vi "NonCoherencyWindowing.vi"() -> ()   [LabVIEW 2009]
uses:
  <vilib>/imath/engines/lvmath2/RunTimeEngine/ErrorHandling/NIMS_Finalize Error.vi
  <vilib>/imath/engines/lvmath2/RunTimeEngine/Parser/MC_Version.vi
  <vilib>/imath/engines/lvmath2/RunTimeEngine/Managers/WorkSpace/UID Generator.vi
  <vilib>/imath/engines/lvmath2/RunTimeEngine/NodeEndStatement/NIMS_NodeEndStatement_Output.vi
  <instcachedir>/0/NIMS_NodeEndStatement_Output_53EC0D466D134D7ABD903AC30B43404B.lvgen/NIMS_NodeEndStatement_Output_53EC0D466D134D7ABD903AC30B43404B_001.vi
  <vilib>/imath/engines/lvmath2/RunTimeEngine/NodeEndStatement/MC_NodeEndStatement_Dispose.vi
  <vilib>/imath/engines/lvmath/Functions/Error Handling/MergeErrorsWrapper.vi
  <vilib>/imathl/engines/lvmath/Functions/Error Handling/Create Error.vi
  <vilib>/imath/engines/lvmath2/RunTimeEngine/RunTimeType/NIMS_RunTimeType_Get Case Value.vi
  <vilib>/imath/engines/lvmath2/RunTimeEngine/Managers/SymbolTable/Read Variable.vi
  <vilib>/imath/engines/lvmath2/RunTimeEngine/CommandStatement/NIMS_CommandStatement_MaskErr.vi
  <vilib>/imath/engines/lvmath2/RunTimeEngine/Managers/SymbolTable/Write Variable.vi
  <vilib>/imath/engines/lvmath2/RunTimeEngine/RunTimeSymbolToken/NIMS_RunTimeSymbolToken_ResolveUDForVariable.vi
  <vilib>/imath/engines/lvmath2/RunTimeEngine/RangeToken/NIMS_NS_Range - 2 inputs.vi
  <vilib>/imath/engines/lvmath2/RunTimeEngine/ArithmeticOperatorToken/NIMS_NS_ArithmeticOperator_rightdivmx.vi
  <vilib>/imath/engines/lvmath2/RunTimeEngine/RunTimeSymbolToken/NIMS_RunTimeSymbolToken_ReadVariable.vi
  <vilib>/imath/engines/lvmath2/RunTimeEngine/ArithmeticOperatorToken/NIMS_NS_ArithmeticOperator_multmx.vi
  <vilib>/imath/engines/lvmath2/RunTimeEngine/RunTimeSymbolToken/NIMS_RunTimeSymbolToken_ResolveSymbol.vi
  <instcachedir>/0/NIMS_RunTimeSymbolToken_ResolveSymbol_94D143D0F28444E2BA7BB87D83E1A664.lvgen/NIMS_RunTimeSymbolToken_ResolveSymbol_94D143D0F28444E2BA7BB87D83E1A664_000.vi
  <vilib>/imath/engines/lvmath2/RunTimeEngine/ArithmeticOperatorToken/NIMS_NS_ArithmeticOperator_plus.vi
  <vilib>/imath/engines/lvmath2/RunTimeEngine/ArithmeticOperatorToken/NIMS_NS_ArithmeticOperator_minus.vi
  <instcachedir>/0/NIMS_RunTimeSymbolToken_ResolveSymbol_94D143D0F28444E2BA7BB87D83E1A664.lvgen/NIMS_RunTimeSymbolToken_ResolveSymbol_94D143D0F28444E2BA7BB87D83E1A664_001.vi
  <vilib>/imath/engines/lvmath2/RunTimeEngine/RunTimeType/NIMS_RunTimeType_From StrictType (excl LVString).vi
  <vilib>/imath/engines/lvmath2/RunTimeEngine/NonStaticBuiltInFunctions/Manual/NIMS_NS_global.vi
  <vilib>/imath/engines/lvmath2/RunTimeEngine/NonStaticBuiltInFunctions/NIMS_NS_cos.vi
  <vilib>/imath/engines/lvmath2/RunTimeEngine/NonStaticBuiltInFunctions/NIMS_NS_fft.vi
  <vilib>/imath/engines/lvmath2/RunTimeEngine/NonStaticBuiltInFunctions/NIMS_NS_abs.vi
  <vilib>/imath/engines/lvmath2/RunTimeEngine/NonStaticBuiltInFunctions/NIMS_NS_log10.vi
  <vilib>/imath/engines/lvmath2/RunTimeEngine/NodeEndStatement/NIMS_NodeEndStatement_Get Vector.vi
  <instcachedir>/0/NIMS_NodeEndStatement_Get Vector_708AE642CFEE4B9892E482CBBBA3A4D6.lvgen/NIMS_NodeEndStatement_Get Vector_708AE642CFEE4B9892E482CBBBA3A4D6_001.vi
  <vilib>/imath/engines/lvmath2/RunTimeEngine/RunTimeType/NIMS_RunTimeType_To Numeric.vi
  <instcachedir>/0/NIMS_RunTimeType_To Numeric_461D4BB0B5AC4C7A80E516929E1870C9.lvgen/NIMS_RunTimeType_To Numeric_461D4BB0B5AC4C7A80E516929E1870C9_000.vi
  <vilib>/imath/engines/lvmath/Plug In/_Char/NIMS_CH_Character 1D to U8 1D.vi
  <instcachedir>/0/NIMS_NodeEndStatement_Get Vector_708AE642CFEE4B9892E482CBBBA3A4D6.lvgen/NIMS_NodeEndStatement_Get Vector_708AE642CFEE4B9892E482CBBBA3A4D6_002.vi
  <vilib>/imath/engines/lvmath/Plug In/_Char/RunTimeType/NIMS_CH_RunTimeType_To Character 2D.vi
  <vilib>/imath/engines/lvmath/Functions/Error Handling/error.ctl
  <vilib>/imath/engines/lvmath2/RunTimeEngine/ArithmeticOperatorToken/NIMS_NS_ArithmeticOperator_times.vi
  <vilib>/imath/engines/lvmath2/RunTimeEngine/ArithmeticOperatorToken/NIMS_NS_ArithmeticOperator_cctranspose.vi
  <vilib>/imath/engines/lvmath2/RunTimeEngine/NonStaticBuiltInFunctions/NIMS_NS_win_hann2.vi
  <vilib>/imath/engines/lvmath2/RunTimeEngine/NonStaticBuiltInFunctions/NIMS_NS_freqzd.vi
  <vilib>/imath/engines/lvmath2/RunTimeEngine/NonStaticBuiltInFunctions/NIMS_NS_win_hamming.vi
  <vilib>/imath/engines/lvmath2/RunTimeEngine/NonStaticBuiltInFunctions/NIMS_NS_win_rect.vi
  <vilib>/imath/engines/lvmath2/RunTimeEngine/Managers/SymbolTable/NIMS_WorkSpace.lvlib
panel:
  in  "Tab Control":enum32{"Input Signals", "Windowing Response"}(tab)
  out "Time":dbl[](graph)=[1.0519999999999998, 0.892635758350692, 0.48671366566360336, -0.014213960529799927, -0.48286399816495823, -0.8332750693454192, -0.9844439089484842, -0.8790173197927672, -0.5425141352910673, -0.07907293537832781, 0.39766710213006506, 0.7950512926839483, 1.0127676392121494, 0.9537752599165119, 0.6072435956998912, 0.0922920759743344, -0.41561505518673614, -0.7885340013883491, -0.9648884833134171, -0.911548116681293, -0.6264833485669233, -0.17599282135085542, 0.31594201614569883, 0.7279199339174797, 0.9717386381220531, 0.9789366799794423, 0.7140755998833661, 0.22979152936681138, -0.32102600764294553, -0.76153026470899, -0.979672712648837, -0.9457238312903217, -0.6821570337182414, -0.25169868445329474, 0.2399555283178424, 0.6689028600572418, 0.9344300816682857, 0.9747853105549835, 0.7654072870023012, 0.3376131259459527, -0.19825451970370167, -0.6793358027763582, -0.9634650376378693, -0.9837135532483375, -0.7508142403449144, -0.33382717711029797, 0.1566403020999526, 0.5966924386654645, 0.8876652145787984, 0.9715292169265111, 0.8206100103361844, 0.44487353719016887, -0.07499320335923955, -0.5870694406395051, -0.9326941295433538, -1.019040372240394, -0.8358834391160587, -0.43566821485006507, 0.07592488783600401, 0.5544251498665185, 0.8704100296507408, 0.964260301096264, 0.8383083974973854, 0.5137376584936127, 0.03499999999999957, -0.48585261295939564, -0.8818652804506516, -1.0229561184206226, -0.8845509930676749, -0.5247145097090272, -0.03421866135883577, 0.46859297497064295, 0.840786779414677, 0.9751969639176659, 0.8614359855640242, 0.5601553978306019, 0.1333879750007619, -0.356995848551684, -0.7952068779929633, -1.0252578021844054, -0.9547362823906638, -0.620110912675251, -0.137507594251358, 0.372068182475295, 0.791142680899002, 0.9993468717462828, 0.9279628829910677, 0.6173563155048777, 0.1802855497563253, -0.28407697645575897, -0.702914526162896, -0.9776488534124683, -0.9933831759695436, -0.7139122080215445, -0.23334898138495994, 0.28978814517635426, 0.7221570337182422, 0.9703821129164357, 0.9663755650482756, 0.7004567661150796, 0.2581711069013682, -0.2223730173404324, -0.6324440323293156, -0.9073207446267804, -0.9820539394221334, -0.7966372182568109, -0.36908259607946664, 0.1722255147849101, 0.6557003844606163, 0.9527237315353941, 0.9994814002292728, 0.78509143650267, 0.36268612299860076, -0.14503930774567764, -0.594528329039942, -0.8856811014773216, -0.9710022598166805, -0.8268249390909151, -0.45949731137287486, 0.05406040835925627, 0.5658950662399057, 0.920493181781949, 1.0203444418805658, 0.8458311373029045, 0.4491073291399612, -0.05639584288440221, -0.528310205810283, -0.8499316903093769]
  out "Frequency Domain":dbl[](graph)=[-36.063010068605344, -35.48013279039274, -34.00368270005921, -32.08344281023172, -29.968400742690303, -27.713180557630817, -25.259324216625465, -22.455608089448322, -18.990832409863973, -14.07794602915972, -4.114913838712823, -3.7403821330415536, -12.946788106870805, -17.080106791999548, -19.72637758714805, -21.54183948254877, -23.16627515506536, -24.401566317457796, -25.443897985258722, -26.343781674957675, -24.226903730320053, -27.839889690043492, -28.476824068317693, -29.059155277051325, -29.599056422316544, -30.110000536672633, -30.614092450790913, -31.1765534431675, -32.358923373450644, -30.386487172294476, -29.468348510203928, -31.912759453430546, -32.26618517164874, -32.57308011024947, -32.85063385246029, -33.10613681596499, -33.343474150812, -33.565060432808615, -33.77256514899041, -33.96723171385923, -34.15003564865244, -34.32177087608298, -34.48310064590985, -34.634589628770996, -34.776725291880645, -34.909932813665826, -35.03458590340212, -35.15101490873227, -35.259513056057415, -35.36034136097869, -35.45373256257553, -35.53989432202372, -35.61901185371619, -35.69125010943872, -35.75675560394464, -35.81565794790601, -35.868071138314555, -35.91409464485639, -35.95381432218219, -35.98730317150038, -36.01462196987916, -36.03581978166229, -36.0509343632001, -36.05999246943212]
  out "Window (time domain)":dbl[][](graph)=[[1.0, 1.0, 1.0, 1.0, 1.0, 1.0, 1.0, 1.0, 1.0, 1.0, 1.0, 1.0, 1.0, 1.0, 1.0, 1.0, 1.0, 1.0, 1.0, 1.0, 1.0, 1.0, 1.0, 1.0, 1.0, 1.0, 1.0, 1.0, 1.0, 1.0, 1.0, 1.0, 1.0, 1.0, 1.0, 1.0, 1.0, 1.0, 1.0, 1.0, 1.0, 1.0, 1.0, 1.0, 1.0, 1.0, 1.0, 1.0, 1.0, 1.0, 1.0, 1.0, 1.0, 1.0, 1.0, 1.0, 1.0, 1.0, 1.0, 1.0, 1.0, 1.0, 1.0, 1.0, 1.0, 1.0, 1.0, 1.0, 1.0, 1.0, 1.0, 1.0, 1.0, 1.0, 1.0, 1.0, 1.0, 1.0, 1.0, 1.0, 1.0, 1.0, 1.0, 1.0, 1.0, 1.0, 1.0, 1.0, 1.0, 1.0, 1.0, 1.0, 1.0, 1.0, 1.0, 1.0, 1.0, 1.0, 1.0, 1.0, 1.0, 1.0, 1.0, 1.0, 1.0, 1.0, 1.0, 1.0, 1.0, 1.0, 1.0, 1.0, 1.0, 1.0, 1.0, 1.0, 1.0, 1.0, 1.0, 1.0, 1.0, 1.0, 1.0, 1.0, 1.0, 1.0, 1.0, 1.0], [0.08000000000000002, 0.0805628485414398, 0.08225001678106098, 0.08505737593545987, 0.08897805592635233, 0.09400246219280656, 0.10011829917074133, 0.10731060038223178, 0.11556176506098892, 0.12485160122438388, 0.13515737508661335, 0.14645386669208266, 0.15871343163286344, 0.17190606869919217, 0.1859994932974579, 0.20095921645601267, 0.21674862922546456, 0.2333290922669115, 0.25066003040887846, 0.2686990319415611, 0.28740195240538674, 0.3067230226199045, 0.326614960688639, 0.34702908770581475, 0.3679154468817952, 0.38922292579571877, 0.4108993814761573, 0.432891768003705, 0.45514626632323235, 0.4776084159481323, 0.500223248234257, 0.5229354208974016, 0.545689353445147, 0.5684293631916387, 0.5910998015224502, 0.6136451900760669, 0.6360103565087342, 0.6581405695104273, 0.6799816727415386, 0.7014802173625158, 0.7225835928321281, 0.7432401556542779, 0.7633993557582885, 0.7830118602033985, 0.8020296739047343, 0.8204062570853257, 0.8380966391667384, 0.8550575288196159, 0.8712474199048162, 0.8866266930458899, 0.9011577125843333, 0.9148049186803513, 0.9275349143337444, 0.9393165471119648, 0.9501209853853384, 0.9599217888828946, 0.9686949733961399, 0.9764190694724346, 0.9830751749543423, 0.9886470012363748, 0.9931209131259411, 0.9964859622109474, 0.9987339136523963, 0.9998592663364182, 0.9998592663364182, 0.9987339136523963, 0.9964859622109474, 0.9931209131259411, 0.9886470012363748, 0.9830751749543423, 0.9764190694724346, 0.9686949733961399, 0.9599217888828946, 0.9501209853853384, 0.9393165471119648, 0.9275349143337444, 0.9148049186803513, 0.9011577125843333, 0.8866266930458899, 0.8712474199048162, 0.8550575288196159, 0.8380966391667384, 0.8204062570853257, 0.8020296739047343, 0.7830118602033985, 0.7633993557582885, 0.7432401556542779, 0.7225835928321281, 0.7014802173625158, 0.6799816727415386, 0.6581405695104273, 0.6360103565087342, 0.6136451900760669, 0.5910998015224502, 0.5684293631916387, 0.545689353445147, 0.5229354208974016, 0.500223248234257, 0.4776084159481323, 0.45514626632323235, 0.432891768003705, 0.4108993814761573, 0.38922292579571877, 0.3679154468817952, 0.34702908770581475, 0.326614960688639, 0.3067230226199045, 0.28740195240538674, 0.2686990319415611, 0.25066003040887846, 0.2333290922669115, 0.21674862922546456, 0.20095921645601267, 0.1859994932974579, 0.17190606869919217, 0.15871343163286344, 0.14645386669208266, 0.13515737508661335, 0.12485160122438388, 0.11556176506098892, 0.10731060038223178, 0.10011829917074133, 0.09400246219280656, 0.08897805592635233, 0.08505737593545987, 0.08225001678106098, 0.0805628485414398, 0.08000000000000002], [0.0005929723795884967, 0.002370483053382111, 0.0053283159624449294, 0.00945945545390292, 0.014754102921297418, 0.021199700045797076, 0.028780958583142835, 0.037479896625674025, 0.047275881253426744, 0.05814567747314048, 0.070063503329095, 0.0830010910550611, 0.09692775412231869, 0.1118104600247129, 0.12761390862810912, 0.14430061589841114, 0.16183100280954865, 0.18016348922055442, 0.19925459249906485, 0.21905903065731985, 0.23952982975603493, 0.2606184353213955, 0.28227482751090444, 0.30444763975492206, 0.3270842805924943, 0.35013105841248787, 0.3735333088041597, 0.3972355242150998, 0.4211814856090132, 0.44531439581106286, 0.46957701422449305, 0.49391179259900125, 0.5182610115288294, 0.5425669173568178, 0.566771859159699, 0.5908184254897182, 0.614649580548245, 0.6382087994683857, 0.6614402023857231, 0.6842886869791809, 0.7067000591676414, 0.7286211616523193, 0.75, 0.7707858659680922, 0.7909294577789764, 0.8103829970583742, 0.829100342160374, 0.8470370976103169, 0.8641507194059579, 0.8804006159271389, 0.895748244214627, 0.9101572013897554, 0.9235933109980301, 0.9360247040719036, 0.9474218947204458, 0.9577578500666184, 0.9670080543662738, 0.975150567156791, 0.9821660752974292, 0.9880379387779634, 0.9927522301869512, 0.9962977677460131, 0.9986661418317757, 0.9998517349225695, 0.9998517349225695, 0.9986661418317757, 0.9962977677460131, 0.9927522301869512, 0.9880379387779634, 0.9821660752974292, 0.975150567156791, 0.9670080543662738, 0.9577578500666184, 0.9474218947204458, 0.9360247040719036, 0.9235933109980301, 0.9101572013897554, 0.895748244214627, 0.8804006159271389, 0.8641507194059579, 0.8470370976103169, 0.829100342160374, 0.8103829970583742, 0.7909294577789764, 0.7707858659680922, 0.75, 0.7286211616523193, 0.7067000591676414, 0.6842886869791809, 0.6614402023857231, 0.6382087994683857, 0.614649580548245, 0.5908184254897182, 0.566771859159699, 0.5425669173568178, 0.5182610115288294, 0.49391179259900125, 0.46957701422449305, 0.44531439581106286, 0.4211814856090132, 0.3972355242150998, 0.3735333088041597, 0.35013105841248787, 0.3270842805924943, 0.30444763975492206, 0.28227482751090444, 0.2606184353213955, 0.23952982975603493, 0.21905903065731985, 0.19925459249906485, 0.18016348922055442, 0.16183100280954865, 0.14430061589841114, 0.12761390862810912, 0.1118104600247129, 0.09692775412231869, 0.0830010910550611, 0.070063503329095, 0.05814567747314048, 0.047275881253426744, 0.037479896625674025, 0.028780958583142835, 0.021199700045797076, 0.014754102921297418, 0.00945945545390292, 0.0053283159624449294, 0.002370483053382111, 0.0005929723795884967]]
  out "Frequency Domain":dbl[][](graph)=[[-36.063010068605344, -35.48013279039274, -34.00368270005921, -32.08344281023172, -29.968400742690303, -27.713180557630817, -25.259324216625465, -22.455608089448322, -18.990832409863973, -14.07794602915972, -4.114913838712823, -3.7403821330415536, -12.946788106870805, -17.080106791999548, -19.72637758714805, -21.54183948254877, -23.16627515506536, -24.401566317457796, -25.443897985258722, -26.343781674957675, -24.226903730320053, -27.839889690043492, -28.476824068317693, -29.059155277051325, -29.599056422316544, -30.110000536672633, -30.614092450790913, -31.1765534431675, -32.358923373450644, -30.386487172294476, -29.468348510203928, -31.912759453430546, -32.26618517164874, -32.57308011024947, -32.85063385246029, -33.10613681596499, -33.343474150812, -33.565060432808615, -33.77256514899041, -33.96723171385923, -34.15003564865244, -34.32177087608298, -34.48310064590985, -34.634589628770996, -34.776725291880645, -34.909932813665826, -35.03458590340212, -35.15101490873227, -35.259513056057415, -35.36034136097869, -35.45373256257553, -35.53989432202372, -35.61901185371619, -35.69125010943872, -35.75675560394464, -35.81565794790601, -35.868071138314555, -35.91409464485639, -35.95381432218219, -35.98730317150038, -36.01462196987916, -36.03581978166229, -36.0509343632001, -36.05999246943212], [-58.449214890565685, -57.99659301664542, -56.830995354748104, -55.31189698579262, -53.7146866380066, -52.24850059037321, -51.290702124199456, -52.56184609062422, -52.14152721463254, -23.812615816221204, -7.165803164294932, -7.1228607660459105, -24.111619061462353, -64.40253961711923, -47.17904359871747, -44.31719208945485, -46.881912664753706, -47.37761953176757, -48.10312057432601, -43.65020997459622, -35.095472401078226, -43.79703893366791, -50.64479328733949, -51.195227399082924, -51.687741149489874, -52.12797936004413, -52.445441805049924, -51.52972015709853, -54.79069186325457, -46.34124538232585, -43.48620172785894, -54.501627772208025, -54.32602334200731, -54.59576780347184, -54.85324775556801, -55.09663588031022, -55.32568812631535, -55.541089024203416, -55.74369836011404, -55.93433737151728, -56.11373989821713, -56.28255011863903, -56.44133216103394, -56.59058141004296, -56.730734708197694, -56.86217890248285, -56.985257841180186, -57.100278077584655, -57.207513535062816, -57.30720934661722, -57.399585037342845, -57.4848371802082, -57.56314162564688, -57.634655382524535, -57.69951821079246, -57.75785397298067, -57.8097717816292, -57.85536697219292, -57.89472192476338, -57.92790675339689, -57.954979877965854, -57.975988490364244, -57.99096892442429, -57.999946936674036], [-83.34386134085403, -79.51898448761983, -74.41497834275134, -69.88171313070012, -65.42745455500169, -60.62260479335387, -55.047430427890205, -48.09810894209579, -38.51683604141908, -21.67308330490058, -7.399057138301478, -7.399587499738757, -21.670243155345588, -38.495537021030735, -47.35192123671943, -50.6774583928388, -55.54580640491036, -64.6462600899097, -68.25108457748827, -42.455394602807644, -36.4363412545581, -42.49225328167863, -78.74873867033841, -82.01933820899842, -85.09168014252842, -89.59436154764377, -85.48350430035154, -65.21919441063662, -50.424823400041134, -48.382494371692786, -45.94777086049274, -52.02671911848568, -86.84510893054434, -91.6763508342159, -94.85726497818345, -97.231719812235, -99.16062599066171, -100.82373560746531, -102.31782811860043, -103.69856120247323, -104.99992144143911, -106.24382814740838, -107.4451318540664, -108.6143395436835, -109.75915966202358, -110.88540368311078, -111.99751880586886, -113.09889679541087, -114.19203697485099, -115.27860489834934, -116.35940747427134, -117.43429276546459, -118.5019751554047, -119.55978282041771, -120.6033247354756, -121.62608093843353, -122.61893597055837, -123.5697061197059, -124.46276183595026, -125.27891621695684, -125.99582393957598, -126.5891666769349, -127.03481151914693, -127.31184145667031]]
  out "Windowed Power Spectrum":cluster{dbl[], dbl[]}[](graph)
  in  "N":dbl=128.0
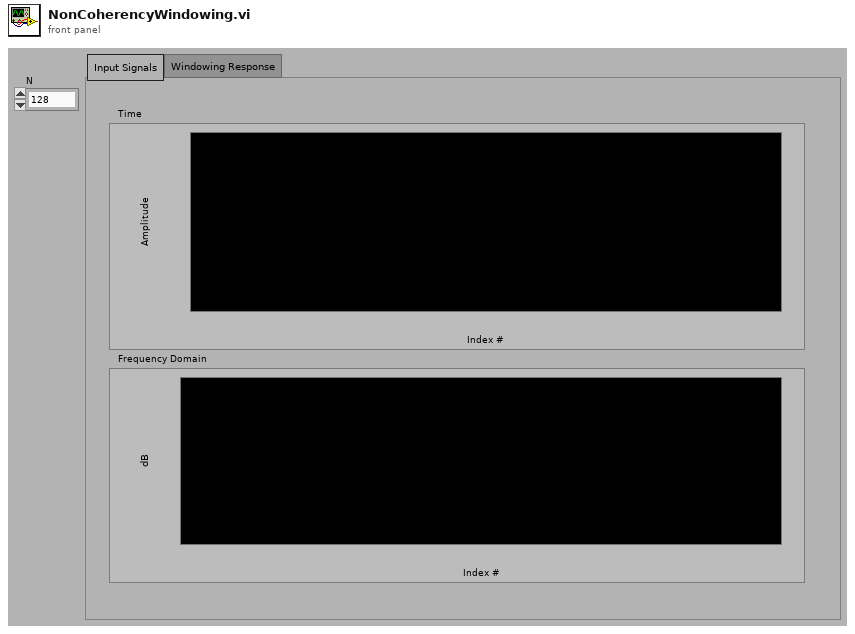
[diagram p1: front panel]
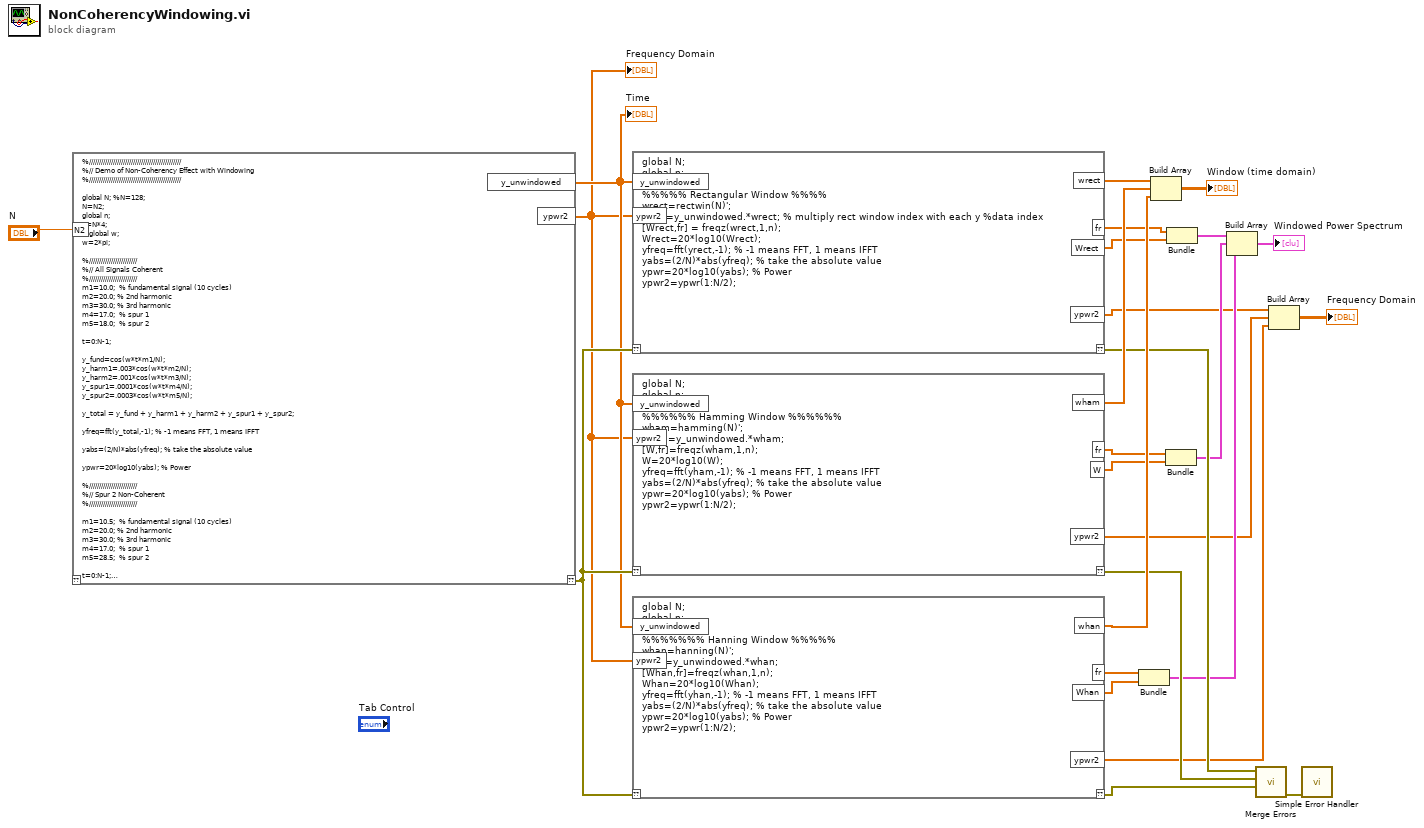
[diagram p0: block diagram]
diagram:
  n1 = mathscript code="%//////////////////////////////////////////////\n%// Demo of Non-Coherency Effect with Windowing\n%//////////////////////////////////////////////\n\nglobal N; %N=128;\nN=N2;\nglobal n; \nn=N*4;\n%global w; \nw=2*pi;\n\n%////////////////////////\n%// All Signals Coherent\n%////////////////////////\nm1=10.0;  % fundamental signal (10 cycles)\nm2=20.0; % 2nd harmonic\nm3=30.0; % 3rd harmonic\nm4=17.0;  % spur 1\nm5=18.0;  % spur 2\n\nt=0:N-1;\n\ny_fund=cos(w*t*m1/N);\ny_harm1=.003*cos(w*t*m2/N);\ny_harm2=.001*cos(w*t*m3/N);\ny_spur1=.0001*cos(w*t*m4/N);\ny_spur2=.0003*cos(w*t*m5/N);\n\ny_total = y_fund + y_harm1 + y_harm2 + y_spur1 + y_spur2;\n\nyfreq=fft(y_total,-1); % -1 means FFT, 1 means IFFT\n\nyabs=(2/N)*abs(yfreq); % take the absolute value\n\nypwr=20*log10(yabs); % Power\n\n%////////////////////////\n%// Spur 2 Non-Coherent\n%////////////////////////\n\nm1=10.5;  % fundamental signal (10 cycles)\nm2=20.0; % 2nd harmonic\nm3=30.0; % 3rd harmonic\nm4=17.0;  % spur 1\nm5=28.5;  % spur 2\n\nt=0:N-1;\n\ny_fund=cos(w*t*m1/N);\ny_harm1=.03*cos(w*t*m2/N);\ny_harm2=.01*cos(w*t*m3/N);\ny_spur1=.005*cos(w*t*m4/N);\ny_spur2=.007*cos(w*t*m5/N);\n\ny_unwindowed = y_fund + y_harm1 + y_harm2 + y_spur1 + y_spur2;\n\n%plot(y_unwindowed); % time domain of all signals\n\n%pause\n\nyfreq=fft(y_unwindowed,-1); % -1 means FFT, 1 means IFFT\nyabs=(2/N)*abs(yfreq); % take the absolute value\nypwr=20*log10(yabs); % Power\nypwr2=ypwr(1:N/2);\n\n%plot(ypwr2);\n\n%pause"("N2"="N") -> ("??"=w21:errorcluster, "y_unwindowed"=w16:dbl[], "ypwr2"=w15:dbl[])  [unwired: 1 in]
  "Time" <- w16
  "Frequency Domain" <- w15
  n2 = mathscript code="global N;\nglobal n; \n\n%%%%% Rectangular Window %%%%\nwrect=rectwin(N)';\nyrect=y_unwindowed.*wrect; % multiply rect window index with each y %data index\n[Wrect,fr] = freqz(wrect,1,n);\nWrect=20*log10(Wrect);\nyfreq=fft(yrect,-1); % -1 means FFT, 1 means IFFT\nyabs=(2/N)*abs(yfreq); % take the absolute value\nypwr=20*log10(yabs); % Power\nypwr2=ypwr(1:N/2);"("??"=w21, "y_unwindowed"=w16, "ypwr2"=w15) -> ("??"=w18:errorcluster, "ypwr2"=w4:dbl[], "wrect"=w25:dbl[], "Wrect"=w13:dbl[], "fr"=w14:dbl[])
  n3 = mathscript code="global N;\nglobal n; \n\n%%%%%% Hamming Window %%%%%%\nwham=hamming(N)';\nyham=y_unwindowed.*wham;\n[W,fr]=freqz(wham,1,n);\nW=20*log10(W);\nyfreq=fft(yham,-1); % -1 means FFT, 1 means IFFT\nyabs=(2/N)*abs(yfreq); % take the absolute value\nypwr=20*log10(yabs); % Power\nypwr2=ypwr(1:N/2);"("??"=w21, "y_unwindowed"=w16, "ypwr2"=w15) -> ("??"=w19:errorcluster, "ypwr2"=w3:dbl[], "wham"=w23:dbl[], "W"=w11:dbl[], "fr"=w12:dbl[])
  n4 = mathscript code="global N;\nglobal n; \n\n%%%%%%% Hanning Window %%%%%\nwhan=hanning(N)';\nyhan=y_unwindowed.*whan;\n[Whan,fr]=freqz(whan,1,n);\nWhan=20*log10(Whan);\nyfreq=fft(yhan,-1); % -1 means FFT, 1 means IFFT\nyabs=(2/N)*abs(yfreq); % take the absolute value\nypwr=20*log10(yabs); % Power\nypwr2=ypwr(1:N/2);"("??"=w21, "y_unwindowed"=w16, "ypwr2"=w15) -> ("??"=w20:errorcluster, "ypwr2"=w2:dbl[], "whan"=w22:dbl[], "Whan"=w6:dbl[], "fr"=w7:dbl[])
  n5 = Bundle(w7, w6) -> (w5:cluster{dbl[], dbl[]})  [unwired: 1 in]
  n6 = Build Array(w25, w23, w22) -> (→"Window (time domain)":dbl[][])
  n7 = Bundle(w12, w11) -> (w8:cluster{dbl[], dbl[]})  [unwired: 1 in]
  n8 = Bundle(w14, w13) -> (w10:cluster{dbl[], dbl[]})  [unwired: 1 in]
  n9 = Build Array(w10, w8, w5) -> (→"Windowed Power Spectrum":cluster{dbl[], dbl[]}[])
  n10 = call <vilib>:"Merge Errors.vi"("error in 3 (no error)"=w20, "error in 2 (no error)"=w19, "error in 1 (no error)"=w18) -> ("error out"=w17:errorcluster)  [unwired: 4 in]
  n11 = Build Array(w4, w3, w2) -> (→"Frequency Domain":dbl[][])
  n12 = call <vilib>:"Simple Error Handler.vi"("error in (no error)"=w17) -> ()  [unwired: 4 in, 5 out]
